vi "potential-field.vi"(11 "IA State Output in":T1={"our_robots"=[], "enemy_robots"=[], "balls"=[], "geometry"={"field_length"=0, "field_width"=0, "goal_width"=0, "goal_depth"=0, "center_circle_radius"=0, "defense_width"=0, "defense_depth"=0, "free_kick_from_defense_dist"=0, "penalty_spot_from_field_line_dist"=0, "penalty_line_from_spot_dist"=0, "half_moon_depth"=0, "half_moon_width"=0}, "IA Judge"={"stage"="", "command"="", "our_goalie_id"=0.0, "enemy_goalie_id"=0.0, "command enum"=enum."Halt", "Time"=enum."Azul"}, "Received Timestamp"=timestamp(0 s since 1904-01-01), "Events"={"Touch"=FALSE, "id touch"=0.0, "Ball out of \nVision"=FALSE, "Ball inside \nGoalie area"=FALSE, "Robot not responding"=FALSE, "Robots responding status"=[1.0, 1.0, 1.0, 1.0, 1.0, 1.0], "Enemy Ball \nPossession"=FALSE, "Id ini Possession"=0.0, "Ball Possesion"=FALSE, "Id Possesion"=0.0}}) -> (3 "IA State Output out":T1={"our_robots"=[], "enemy_robots"=[], "balls"=[], "geometry"={"field_length"=0, "field_width"=0, "goal_width"=0, "goal_depth"=0, "center_circle_radius"=0, "defense_width"=0, "defense_depth"=0, "free_kick_from_defense_dist"=0, "penalty_spot_from_field_line_dist"=0, "penalty_line_from_spot_dist"=0, "half_moon_depth"=0, "half_moon_width"=0}, "IA Judge"={"stage"="", "command"="", "our_goalie_id"=0.0, "enemy_goalie_id"=0.0, "command enum"=enum."Halt", "Time"=enum."Azul"}, "Received Timestamp"=timestamp(0 s since 1904-01-01), "Events"={"Touch"=FALSE, "id touch"=0.0, "Ball out of \nVision"=FALSE, "Ball inside \nGoalie area"=FALSE, "Robot not responding"=FALSE, "Robots responding status"=[1.0, 1.0, 1.0, 1.0, 1.0, 1.0], "Enemy Ball \nPossession"=FALSE, "Id ini Possession"=0.0, "Ball Possesion"=FALSE, "Id Possesion"=0.0}})   [LabVIEW 2017]
uses:
  Core/AI Input.ctl
  Core/AI Robot.ctl
  Intel/Functions Enum.ctl
  Intel/AttackerStates.ctl
  Path Planning/RRT/PathDests.ctl
  Path Planning/RRT/PathDest.ctl
  Core/AI Ball.ctl
  Core/Field Size.ctl
  Core/AI Judge.ctl
  Intel/Command Enum.ctl
  Util/Events/Events.ctl
  <vilib>/Analysis/_algsub.llb/Vector Norm Type.ctl
  <vilib>/Analysis/_algsub.llb/Real Vector Norm.vi
  <vilib>/Analysis/coordinate.llb/2D Cartesian Coordinate Rotation (Scalar).vi
  <vilib>/Analysis/NI_AALPro.lvlib
panel:
  in  "influence radius":dbl=500.0 format="%#_13g"
  in  "multiplier":dbl(slide)=1.0 scale=0.0..10.0
  in  "dist to nullify pot field":dbl=800.0 format="%#_13g"
  in  "min dist to reduce":dbl=500.0 format="%#_13g"
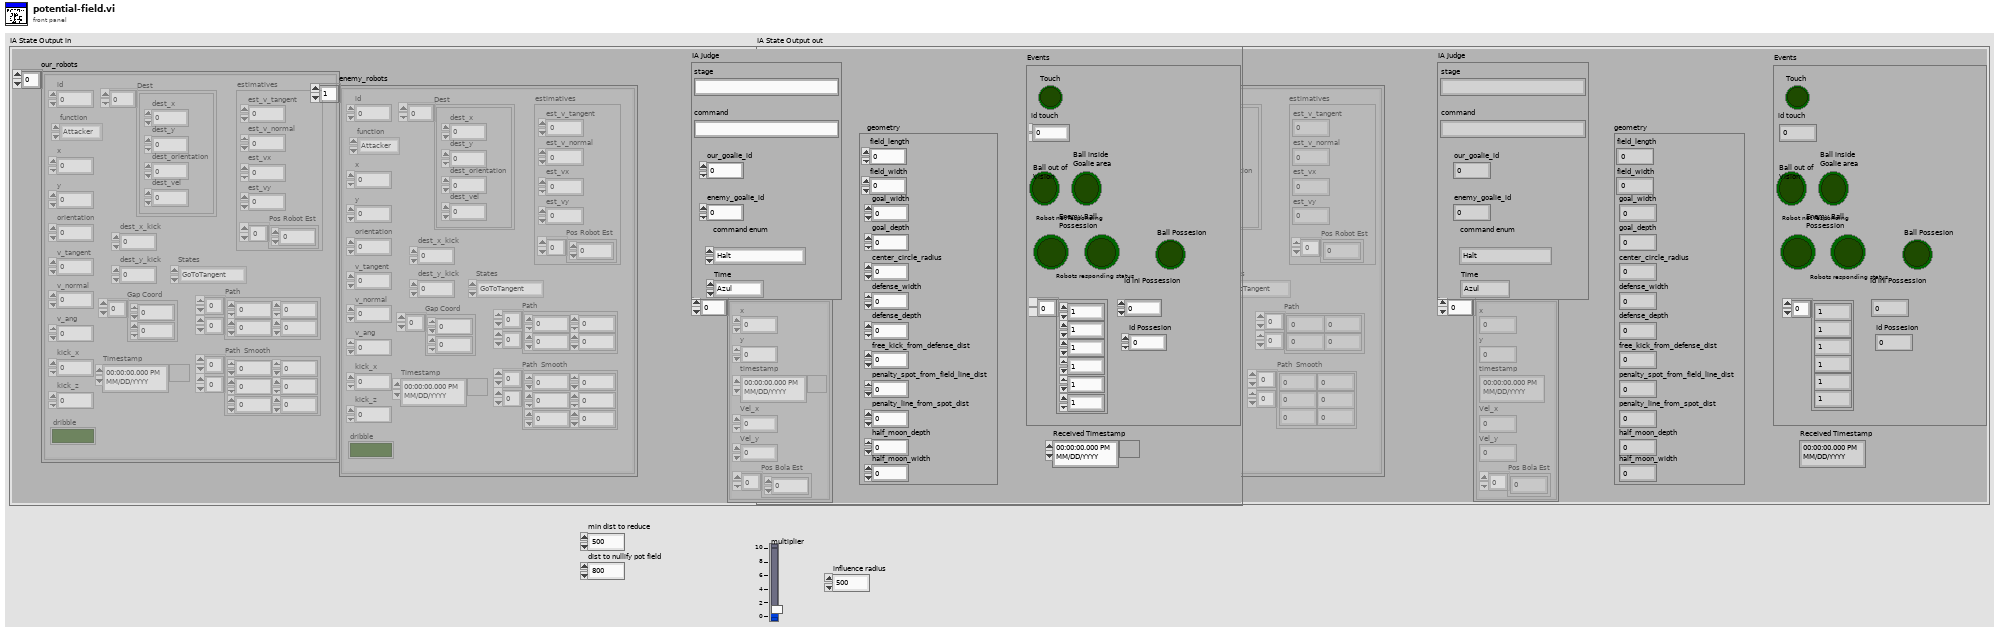
[diagram p1: front panel]
types:
  T1 = typedef "AI Input.ctl" = cluster{"our_robots":T2[], "enemy_robots":T2[], "balls":T7[], "geometry":T8, "IA Judge":T9, "Received Timestamp":timestamp, "Events":T11}
  T2 = typedef "AI Robot.ctl" = cluster{"id":u32, "function":T3, "x":dbl, "y":dbl, "orientation":dbl, "v_tangent":dbl, "v_normal":dbl, "v_ang":dbl, "kick_x":dbl, "kick_z":dbl, "dribble":bool, "Timestamp":timestamp, "estimatives":cluster{"est_v_tangent":dbl, "est_v_normal":dbl, "est_vx":dbl, "est_vy":dbl, "Pos Robot Est":dbl[]}, "dest_x_kick":dbl, "dest_y_kick":dbl, "Gap Coord":dbl[], "States":T4, "Path ":dbl[][], "Path  Smooth":dbl[][], "Dest":T5}
  T3 = typedef "Functions Enum.ctl" = enum16{"Attacker", "Goalie", "Defender", "Striker", "Goto 0", "Dummy", "Kicker", "ZigZag"}
  T4 = typedef "AttackerStates.ctl" = enum16{"Pass", "GoToTangent", "BallGetting", "GoToKick", ""}
  T5 = typedef "PathDests.ctl" = T6[]
  T6 = typedef "PathDest.ctl" = cluster{"dest_x":dbl, "dest_y":dbl, "dest_orientation":dbl, "dest_vel":dbl}
  T7 = typedef "AI Ball.ctl" = cluster{"x":dbl, "y":dbl, "timestamp":timestamp, "Vel_x":dbl, "Vel_y":dbl, "Pos Bola Est":dbl[]}
  T8 = typedef "Field Size.ctl" = cluster{"field_length":u32, "field_width":u32, "goal_width":u32, "goal_depth":u32, "center_circle_radius":u32, "defense_width":u32, "defense_depth":u32, "free_kick_from_defense_dist":u32, "penalty_spot_from_field_line_dist":u32, "penalty_line_from_spot_dist":u32, "half_moon_depth":u32, "half_moon_width":u32}
  T9 = typedef "AI Judge.ctl" = cluster{"stage":string, "command":string, "our_goalie_id":dbl, "enemy_goalie_id":dbl, "command enum":T10, "Time":enum16{"Azul", "Amarelo"}}
  T10 = typedef "Command Enum.ctl" = enum16{"Halt", "Stop", "Force Start", "PKA Normal Start", "Prepare Kickoff Ally", "PKE Normal Start", "Prepare Kickoff Enemy", "Prepare Penalty Ally", "PPA Normal Start", "Prepare Penalty Enemy", "PPE Normal Start", "Direct Free Enemy", "Direct Free Ally", "Indirect Free Enemy", "Indirect Free Ally", "Timeout Enemy", "Timeout Ally", "Goal Enemy", "Goal Ally", "Ball Placement Enemy", "Ball Placement Ally", "Normal Half Time", "Extra Time Break", "Extra Half Time", "None", "Post Game"}
  T11 = typedef "Events.ctl" = cluster{"Touch":bool, "id touch":dbl, "Ball out of \nVision":bool, "Ball inside \nGoalie area":bool, "Robot not responding":bool, "Robots responding status":dbl[], "Enemy Ball \nPossession":bool, "Id ini Possession":dbl, "Ball Possesion":bool, "Id Possesion":dbl}
  T12 = typedef "NI_AALPro.lvlib/Vector Norm Type.ctl" = u16
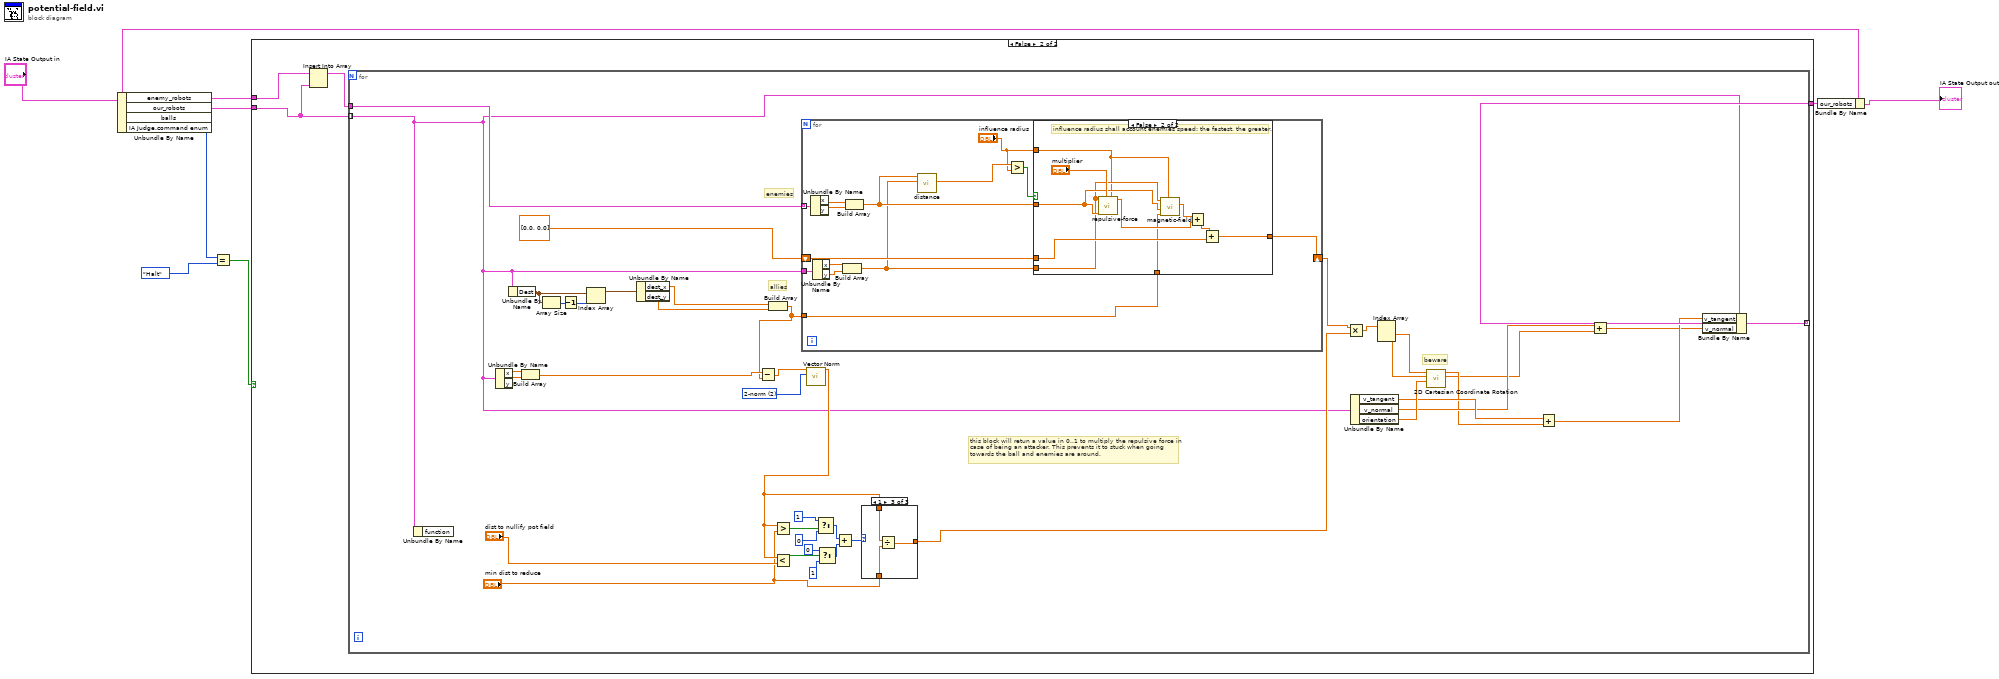
[diagram p0: block diagram]
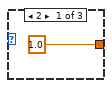
[diagram p3: hidden frame]
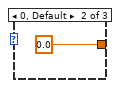
[diagram p4: hidden frame]
diagram:
  n1 = Unbundle By Name("IA State Output in") -> ("enemy_robots"=w8:T2[], "our_robots"=w7:T2[], "IA Judge.command enum"=w3:T10)  [unwired: 1 out]
  n2 = Equal?(x=w3, y=Command_Enum."Halt") -> (x = y?=w1:bool)
  n3 = case shown="False" w1 {
    tunnel: w8 -> [_ w12]
    tunnel: w7 -> [w9 w11]
    tunnel: [w9 w13] -> w6
    frame True {
    }
    frame False {
      n4 = Insert Into Array(array=w12, new element=w11) -> (w10:T2[])  [unwired: 1 in]
      n5 = for {
        tunnel: w10 -> [w53]
        tunnel: w11 -> [w32] mode=indexing
        tunnel: [w43] -> w13 mode=indexing
        w34 = T12 2 items=["1-norm"=1, "2-norm"=2, "Inf-norm"=3, "-Inf-norm"=4, "User Defined"=5] ("norm type")
        # "allies"
        # "enemies"
        # "this block will retun a value in 0..1 to multiply the repulsive force in\ncase of being an attacker. This prevents it to stuck when going \ntowards the ball and enemies are around."
        # "beware"
        n6 = Unbundle By Name(w32) -> ()  [unwired: 1 out]
        n7 = Unbundle By Name(w32) -> ("x"=w38:dbl, "y"=w37:dbl)
        n8 = Unbundle By Name(w32) -> ("Dest"=w16:T5)
        n9 = Build Array(w38, w37) -> (w36:dbl[])
        n10 = Array Size(array=w16) -> (size(s)=w19:i32)
        n11 = Decrement(x=w19) -> (x-1=w18:i32)
        n12 = Index Array(array=w16, index=w18) -> (element=w17:T6)
        n13 = Unbundle By Name(w17) -> ("dest_x"=w15:dbl, "dest_y"=w14:dbl)
        n14 = Build Array(w15, w14) -> (w31:dbl[])
        n15 = Subtract(x=w36, y=w31) -> (x-y=w35:dbl[])
        n16 = for {
          tunnel: w53 -> [w72] mode=indexing
          tunnel: w32 -> [w65]
          shift-right: [w66] -> w41
          shift-left: dbl[] [0.0, 0.0] -> [w67]
          tunnel: w31 -> [w62]
          n17 = Unbundle By Name(w72) -> ("x"=w71:dbl, "y"=w70:dbl)
          n18 = Unbundle By Name(w65) -> ("x"=w69:dbl, "y"=w68:dbl)
          n19 = Build Array(w69, w68) -> (w63:dbl[])
          n20 = Build Array(w71, w70) -> (w64:dbl[])
          n21 = call "distance.vi"("target pos"=w63, "obj pos"=w64) -> ("sqrt(x)"=w61:dbl)  [unwired: 9 in]
          n22 = Greater?(x=w61, y="influence radius") -> (0:w59:bool)
          n23 = case shown="False" w59 {
            tunnel: w67 -> [w73 w83]
            tunnel: [w73 w82] -> w66
            tunnel: w64 -> [_ w77]
            tunnel: w63 -> [_ w76]
            tunnel: w62 -> [_ w75]
            tunnel: "influence radius" -> [_ w74]
            frame True {
            }
            frame False {
              # "influence radius shall account enemies speed: the fastest, the greater."
              n24 = call "repulsive-force.vi"("influence radius"=w74, "multiplier"="multiplier", "obstacle pos"=w77, "agent pos"=w76) -> ("force"=w80:dbl[])  [unwired: 6 in, 1 out]
              n25 = call "magnetic-field.vi"("enemy influence radius"=w74, "goal pos"=w75, "enemy pos"=w77, "ally pos"=w76) -> ("magnetic force"=w81:dbl[])  [unwired: 7 in]
              n26 = Add(x=w81, y=w80) -> (x+y=w79:dbl[])
              n27 = Add(x=w79, y=w83) -> (x+y=w82:dbl[])
            }
          }
        }
        n28 = call-poly <vilib>:"Vector Norm.vi"("norm type"=w34, "Input Vector"=w35) -> ("norm"=w33:dbl)  [unwired: 8 in, 1 out]
        n29 = Less?(x=w33, y="dist to nullify pot field") -> (x < y?=w27:bool)
        n30 = Greater?(x=w33, y="min dist to reduce") -> (0:w28:bool)
        n31 = Select(t=1, s=w28, f=0) -> (s? t:f=w29:i32)
        n32 = Select(t=0, s=w27, f=1) -> (s? t:f=w30:i32)
        n33 = Add(x=w29, y=w30) -> (x+y=w21:i32)
        n34 = case shown="1" w21 {
          tunnel: [1.0 0.0 w56] -> w40
          tunnel: w33 -> [_ _ w58]
          tunnel: "min dist to reduce" -> [_ _ w57]
          frame 2 {
          }
          frame 0, Default {
          }
          frame 1 {
            n35 = Divide(x=w58, y=w57) -> (x/y=w56:dbl)
          }
        }
        n36 = Multiply(x=w41, y=w40) -> (x*y=w39:dbl[])
        n37 = Unbundle By Name(w32) -> ("v_tangent"=w49:dbl, "v_normal"=w48:dbl, "orientation"=w50:dbl)
        n38 = Index Array(array=w39) -> (element #1=w52:dbl, element #2=w51:dbl)  [unwired: 2 in]
        n39 = call-poly <vilib>:"2D Cartesian Coordinate Rotation.vi"("theta"=w50, "y"=w51, "x"=w52) -> ("y out"=w46:dbl, "x out"=w47:dbl)  [unwired: 6 in, 1 out]
        n40 = Add(x=w49, y=w47) -> (x+y=w45:dbl)
        n41 = Add(x=w48, y=w46) -> (x+y=w44:dbl)
        n42 = Bundle By Name(cluster=w32, "v_tangent"=w45, "v_normal"=w44) -> (w43:T2)
      }
    }
  }
  n43 = Bundle By Name(cluster="IA State Output in", "our_robots"=w6) -> (→"IA State Output out":T1)
